vi "TankCommandProcess.vi"(10 "Sensor Cluster":T6, 11 "Command":T8) -> (1 "Non PID Drive Values":T3, 2 "PID Values":T4, 3 "PID Ranges":T1)   [LabVIEW 2017]
uses:
  <userlib>/836-Library/Drive/Drive_Code_V2/Drive_Code_Support/Command_Sends/Drive_Code_Command_Type.ctl
  <userlib>/836-Library/Drive/Drive_Code_V2/Drive_Code_Support/Command_Sends/Drive_Code_Command_List.ctl
  <userlib>/836-Library/Drive/Drive_Code_V2/Drive_Code_Support/SensorTypedefs/Sensor_Cluster.ctl
  <userlib>/836-Library/Drive/Drive_Code_V2/Drive_Code_Support/SensorTypedefs/Camera_Cluster.ctl
  <userlib>/836-Library/Drive/Drive_Code_V2/Drive_Code_Support/PidClusters/DrivePidInputs.ctl
  <userlib>/836-Library/Drive/Drive_Code_V2/Drive_Code_Support/PidClusters/PidInputs.ctl
  <userlib>/836-Library/Drive/Drive_Code_V2/Drive_Code_Support/DriveTrains/Drive_Values.ctl
  <userlib>/836-Library/Drive/Drive_Code_V2/Drive_Code_Support/PidClusters/DrivePidRange.ctl
  <userlib>/836-Library/Drive/Drive_Code_V2/Drive_Code_Support/PidClusters/PidRange.ctl
  <userlib>/836-Library/Drive/Drive_Code_V2/Drive_Code_Support/Command_Sends/CommandTypeInfo/TankDriveParam.ctl
  <userlib>/836-Library/Drive/Drive_Code_V2/Drive_Code_Support/Command_Sends/CommandTypeInfo/DriveContinuousParam.ctl
  <userlib>/836-Library/Drive/Drive_Code_V2/Drive_Code_Support/Command_Sends/CommandTypeInfo/AngleInfo.ctl
  <userlib>/836-Library/Drive/Drive_Code_V2/Drive_Code_Support/Command_Sends/CommandTypeInfo/TurnParam.ctl
  <userlib>/836-Library/Drive/Drive_Code_V2/Drive_Code_Support/Command_Sends/CommandTypeInfo/DriveDistanceParam.ctl
  <userlib>/836-Library/Drive/Drive_Code_V2/Drive_Code_Support/Command_Sends/CommandTypeInfo/DistanceInfo.ctl
  <userlib>/836-Library/Drive/Drive_Code_V2/Drive_Code_Support/Command_Sends/CommandTypeInfo/HoldPositionParam.ctl
  <userlib>/836-Library/Drive/Drive_Code_V2/Drive_Code_Support/Command_Sends/CommandTypeInfo/HoldYawParam.ctl
  <userlib>/836-Library/Drive/Drive_Code_V2/Drive_Code_Support/Command_Sends/CommandTypeInfo/FollowCameraparam.ctl
  <userlib>/836-Library/Drive/Drive_Code_V2/Drive_Code_Support/Command_Sends/CommandTypeInfo/TurnToCameraParam.ctl
  <userlib>/836-Library/Drive/Drive_Code_V2/Drive_Code_Support/Command_Sends/CommandTypeInfo/ApproachCameraParam.ctl
  <userlib>/836-Library/Drive/Drive_Code_V2/Drive_Code_Support/Command_Sends/CommandTypeInfo/CheesyDriveParam.ctl
panel:
  in  "Quick Turn Deadzone":dbl(knob)=0.05 scale=0.0..0.1
  # "I/O"
  # "Configuration Values"
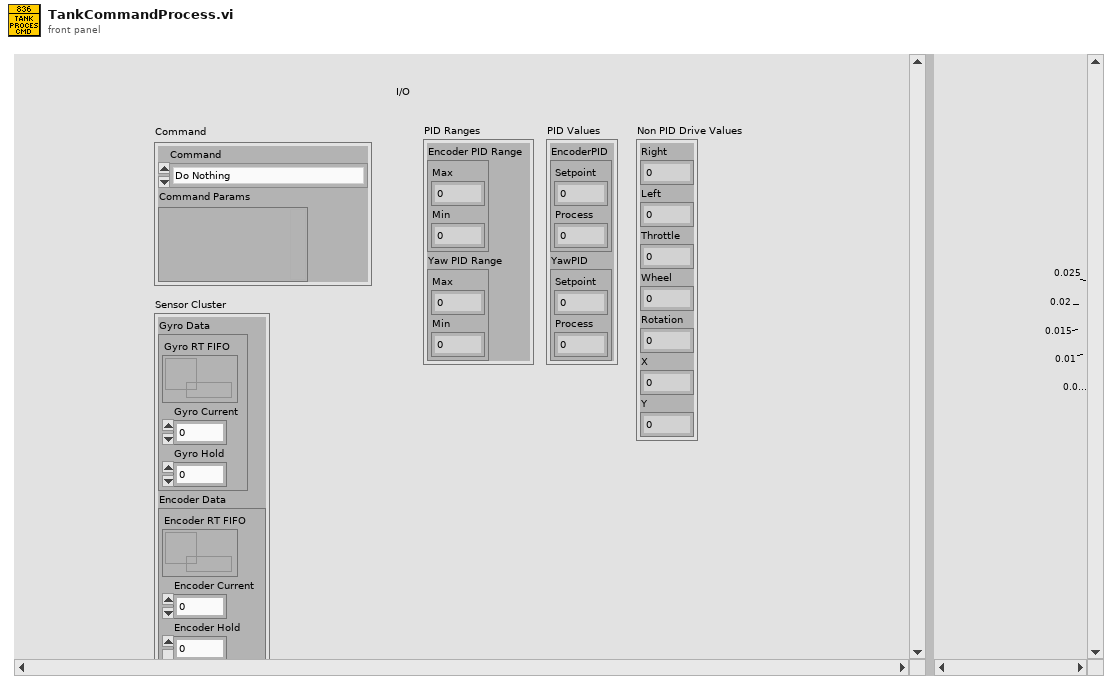
[diagram p1: front panel]
types:
  T1 = typedef "DrivePidRange.ctl" = cluster{"Encoder PID Range":T2, "Yaw PID Range":T2}
  T2 = typedef "PidRange.ctl" = cluster{"Max":dbl, "Min":dbl}
  T3 = typedef "Drive_Values.ctl" = cluster{"Right":dbl, "Left":dbl, "Throttle":dbl, "Wheel":dbl, "Rotation":dbl, "X":dbl, "Y":dbl}
  T4 = typedef "DrivePidInputs.ctl" = cluster{"EncoderPID":T5, "YawPID":T5}
  T5 = typedef "PidInputs.ctl" = cluster{"Setpoint":dbl, "Process":dbl}
  T6 = typedef "Sensor_Cluster.ctl" = cluster{"Gyro Data":cluster{"Gyro RT FIFO":refnum<k33>, "Gyro Current":dbl, "Gyro Hold":dbl}, "Encoder Data":cluster{"Encoder RT FIFO":refnum<k33>, "Encoder Current":dbl, "Encoder Hold":dbl}, "Camera Data":cluster{"Camera RT FIFO":refnum<k33>, "Camera Current":T7}}
  T7 = typedef "Camera_Cluster.ctl" = cluster{" Angle":dbl, "Valid":bool}
  T8 = typedef "Drive_Code_Command_Type.ctl" = cluster{"Command":T9, "Command Params":variant}
  T9 = typedef "Drive_Code_Command_List.ctl" = enum16{"Do Nothing", "Tank Drive", "Drive Continuous", "Turn", "Drive Distance", "Hold Position", "Hold Yaw", "Follow Camera", "Turn to Camera", "Approach Camera", "PID Update", "Cheesy Drive", "Update Period", "Update PID Inversions"}
  T10 = typedef "TankDriveParam.ctl" = cluster{"Left":dbl, "Right":dbl}
  T11 = typedef "DriveContinuousParam.ctl" = cluster{"Max Turn Power":dbl, "Angle To Drive At":T12, "Foward Power":dbl}
  T12 = typedef "AngleInfo.ctl" = cluster{"Angle":dbl, "Angle Absolute?":bool}
  T13 = typedef "TurnParam.ctl" = cluster{"Max Power":dbl, "Angle To Turn To":T12}
  T14 = typedef "DriveDistanceParam.ctl" = cluster{"Max Turn Power":dbl, "Distance To Drive":T15, "Angle To Drive At":T12, "Max Forward Power":dbl}
  T15 = typedef "DistanceInfo.ctl" = cluster{"Distance":dbl, "Distance Absolute?":bool}
  T16 = typedef "HoldPositionParam.ctl" = cluster{"Max Turn Power":dbl, "Max Forward Power":dbl}
  T17 = typedef "HoldYawParam.ctl" = cluster{"Max Turn Power":dbl, "Forward Power":dbl}
  T18 = typedef "FollowCameraparam.ctl" = cluster{"Max Turn Power":dbl, "Forward Power":dbl}
  T19 = typedef "TurnToCameraParam.ctl" = cluster{"Max Turn Power":dbl}
  T20 = typedef "ApproachCameraParam.ctl" = cluster{"Max Turn Power":dbl, "Distance To Drive":T15, "Max Forward Power":dbl}
  T21 = typedef "CheesyDriveParam.ctl" = cluster{"Throttle":dbl, "Wheel":dbl}
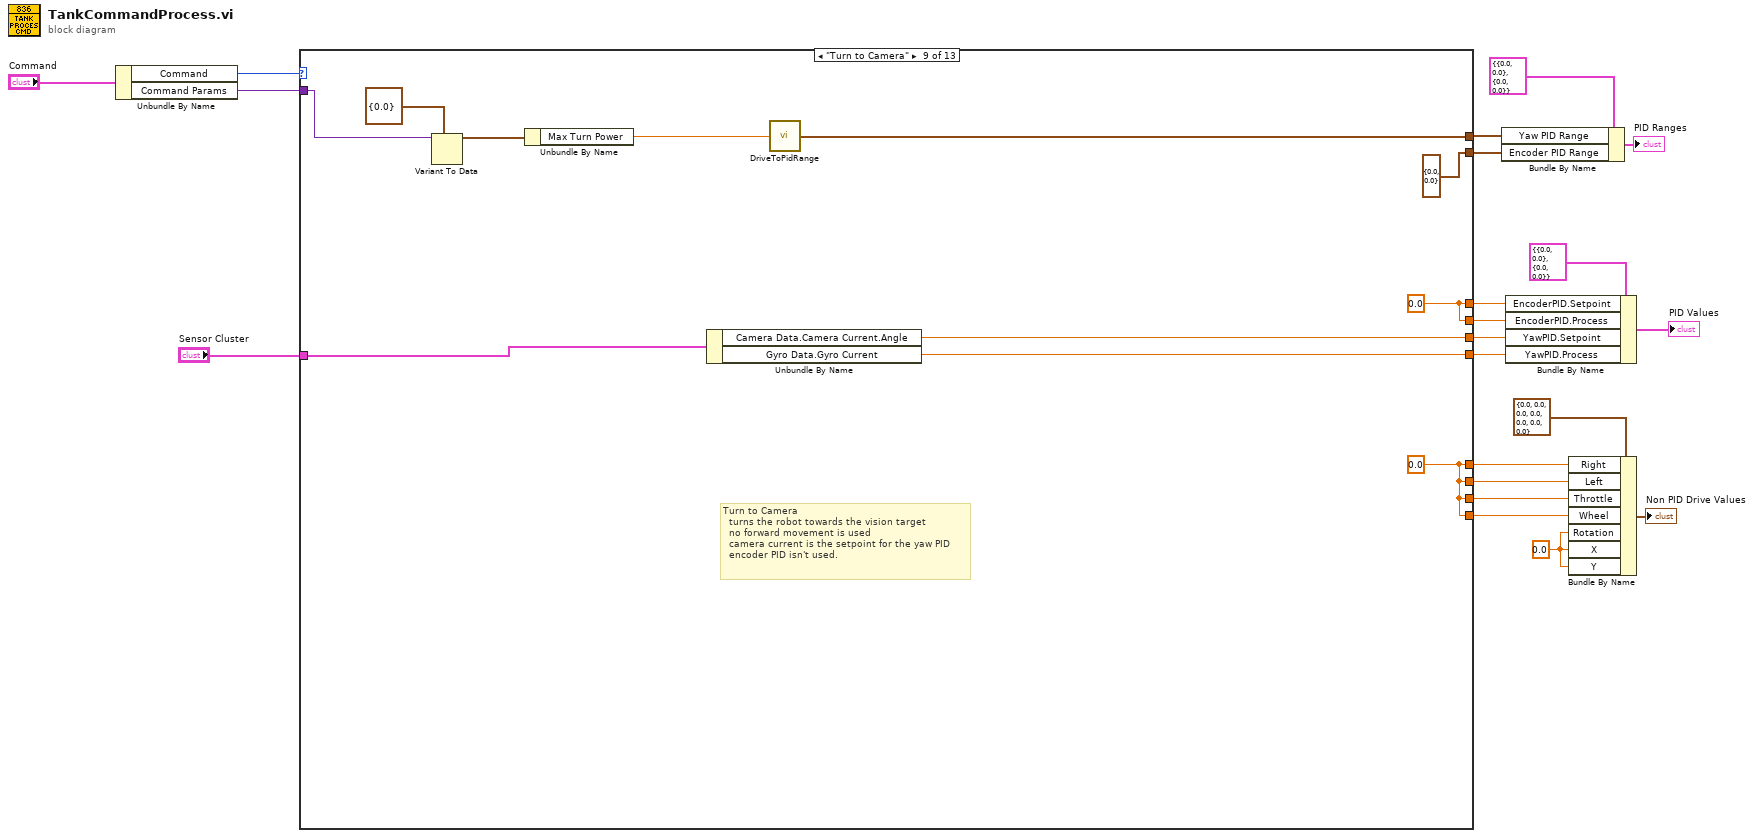
[diagram p0: block diagram]
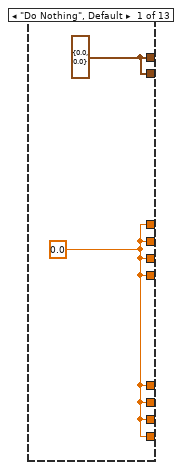
[diagram p2: hidden frame]
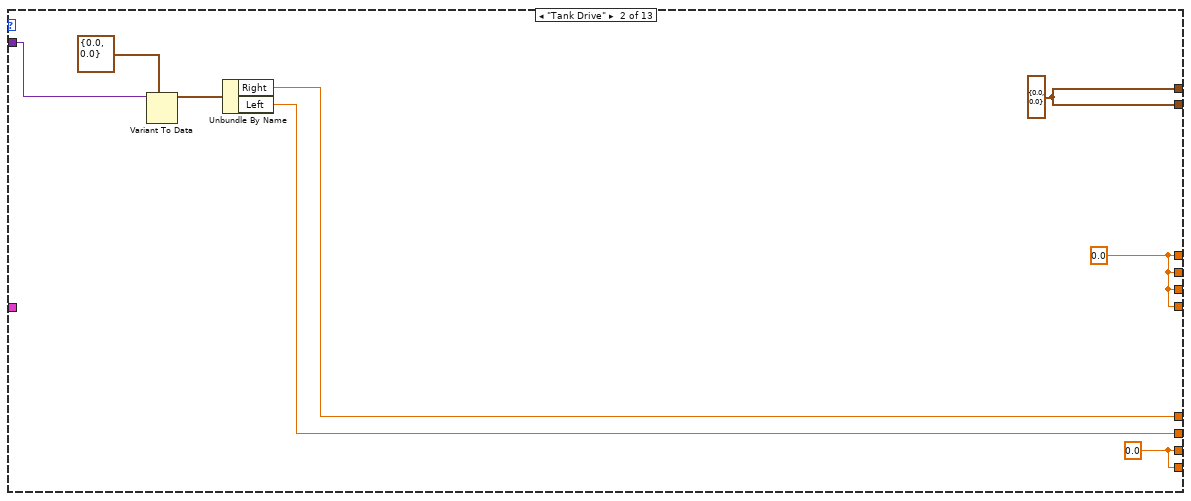
[diagram p3: hidden frame]
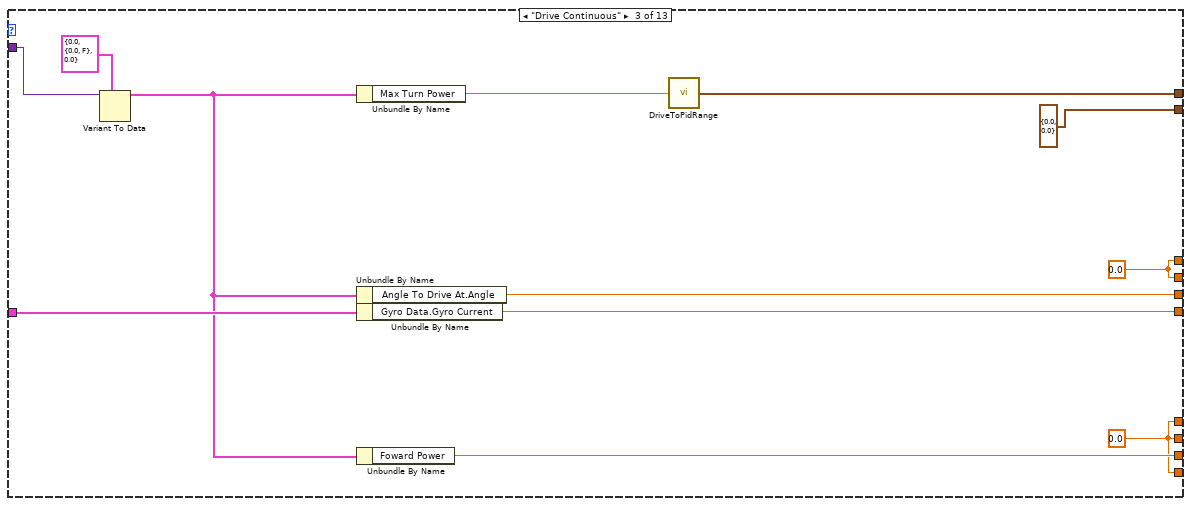
[diagram p4: hidden frame]
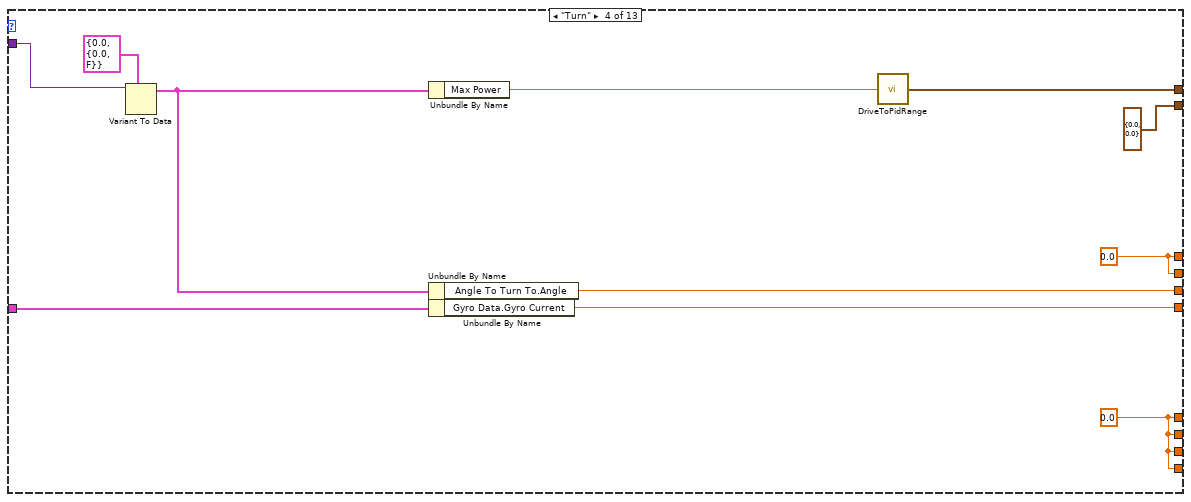
[diagram p5: hidden frame]
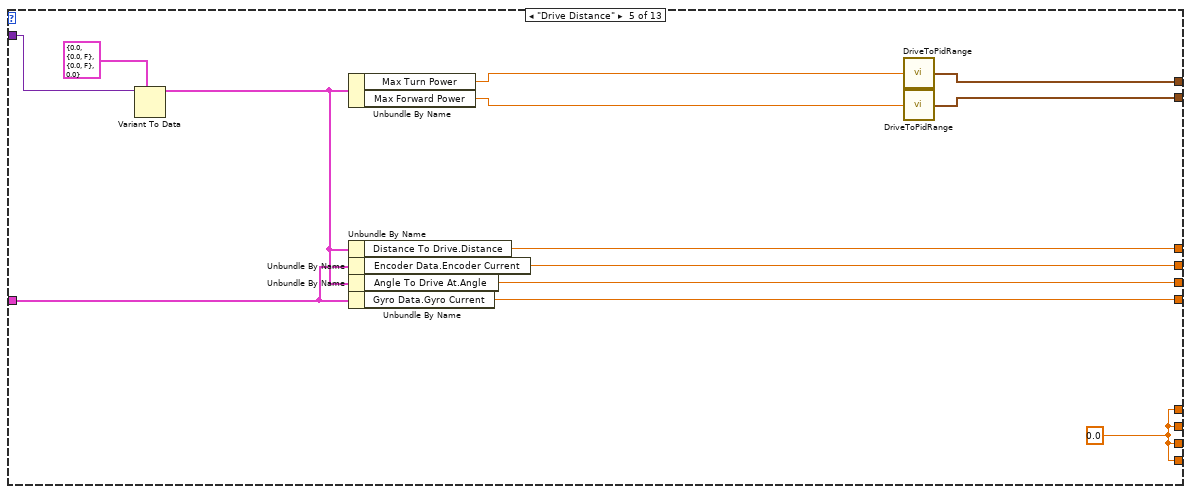
[diagram p6: hidden frame]
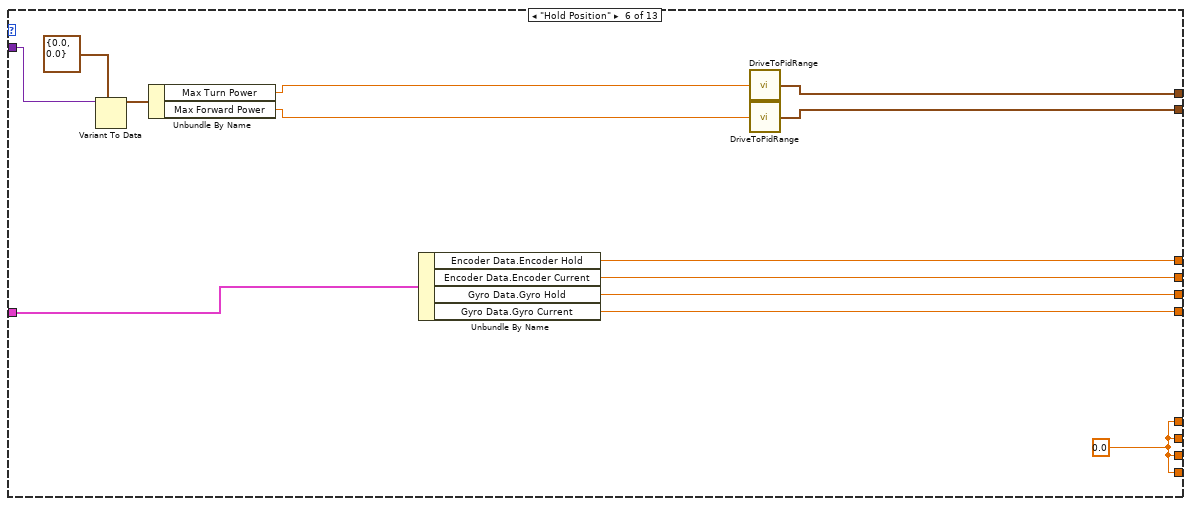
[diagram p7: hidden frame]
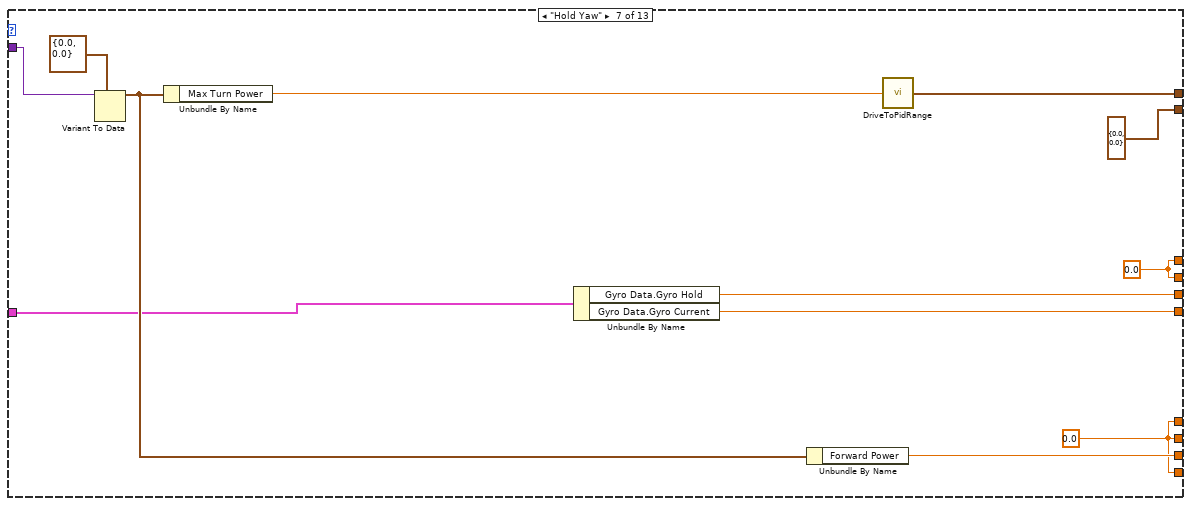
[diagram p8: hidden frame]
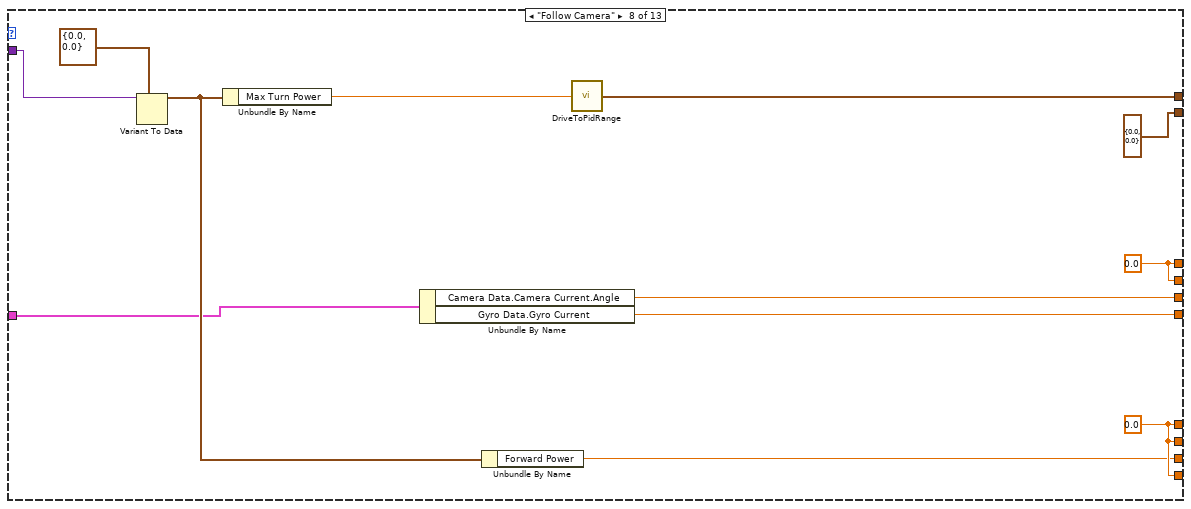
[diagram p9: hidden frame]
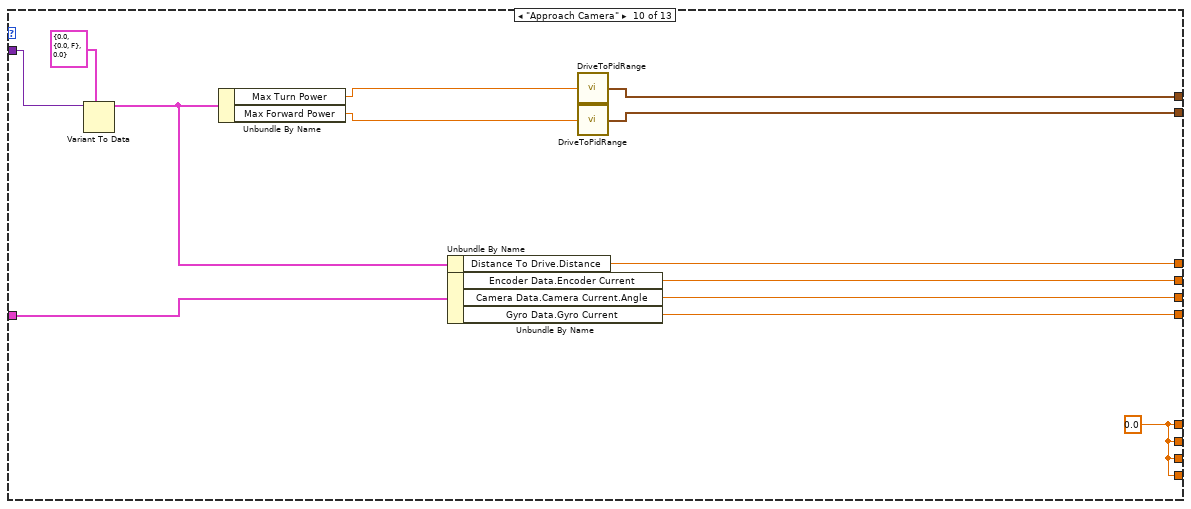
[diagram p10: hidden frame]
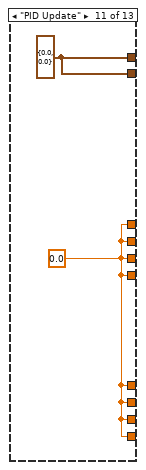
[diagram p11: hidden frame]
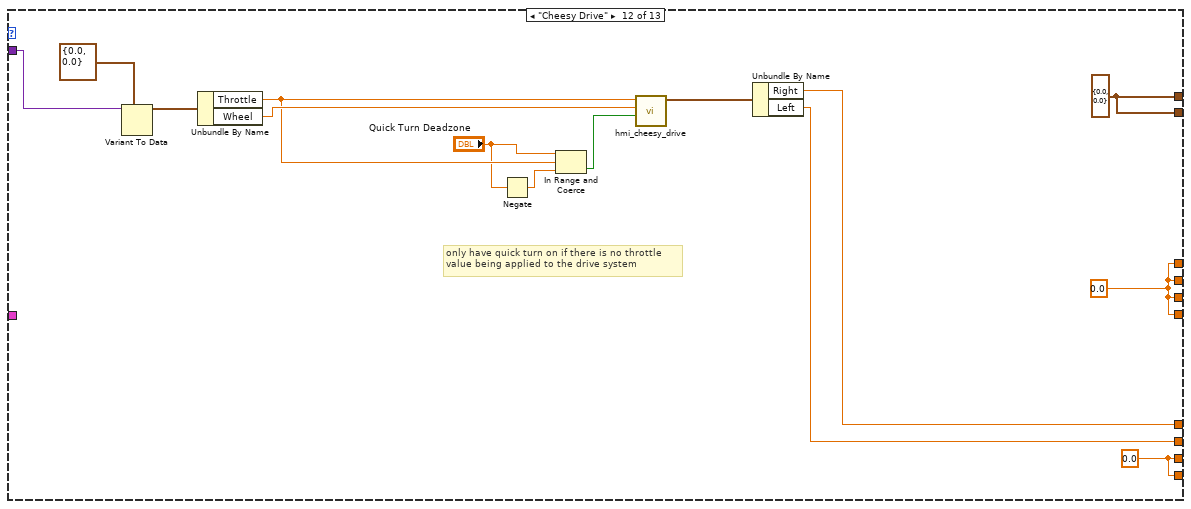
[diagram p12: hidden frame]
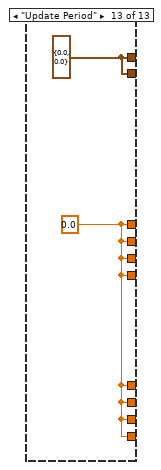
[diagram p13: hidden frame]
diagram:
  w8 = 0.0 ("Rotation")
  n1 = Unbundle By Name("Command") -> ("Command"=w20:T9, "Command Params"=w19:variant)
  n2 = case shown="\"Turn to Camera\"" w20 {
    tunnel: w19 -> [_ w30 w42 w51 w67 w80 w92 w104 w115 w128 _ w143 _]
    tunnel: "Sensor Cluster" -> [_ _ w43 w47 w60 w72 w83 w95 w107 w120 _ _ _]
    tunnel: [w22 w31 w36 w53 w59 w71 w87 w99 w108 w119 w129 w144 w145] -> w16
    tunnel: [w22 w31 w36 w53 w58 w70 w87 w99 w108 w118 w129 w144 w145] -> w15
    tunnel: [w22 w31 w38 w44 w57 w69 w82 w94 w106 w117 w129 w144 w145] -> w14
    tunnel: [w22 w31 w37 w46 w56 w68 w81 w93 w105 w116 w129 w144 w145] -> w13
    tunnel: [w22 w27 w33 w54 w55 w73 w88 w98 w109 w122 w129 w139 w145] -> w10
    tunnel: [w22 w26 w33 w54 w55 w73 w88 w98 w109 w122 w129 w138 w145] -> w9
    tunnel: [w23 w25 w40 w49 w63 w74 w85 w101 w111 w124 w130 w132 w146] -> w3
    tunnel: [w22 w24 w34 w54 w55 w73 w89 w96 w109 w122 w129 w131 w145] -> w6
    tunnel: [w22 w24 w33 w54 w55 w73 w88 w98 w109 w122 w129 w131 w145] -> w5
    tunnel: [w23 w25 T2 {"Max"=0.0, "Min"=0.0} ("PID Range") T2 {"Max"=0.0, "Min"=0.0} ("PID Range") w62 w75 T2 {"Max"=0.0, "Min"=0.0} ("PID Range") T2 {"Max"=0.0, "Min"=0.0} ("PID Range") T2 {"Max"=0.0, "Min"=0.0} ("PID Range") w123 w130 w132 w146] -> w2
    frame "Do Nothing", Default {
      w23 = T2 {"Max"=0.0, "Min"=0.0} ("PID Range")
      w22 = 0.0
    }
    frame "Tank Drive" {
      w24 = 0.0 ("Encoder Hold")
      w25 = T2 {"Max"=0.0, "Min"=0.0} ("PID Range")
      w31 = 0.0
      n3 = Variant To Data(type=T10 {"Left"=0.0, "Right"=0.0} ("Tank Drive Param"), Variant=w30) -> (data=w28:T10)  [unwired: 1 in, 1 out]
      n4 = Unbundle By Name(w28) -> ("Right"=w27:dbl, "Left"=w26:dbl)
    }
    frame "Drive Continuous" {
      w33 = 0.0
      w36 = 0.0
      n5 = Variant To Data(type=T11 {"Max Turn Power"=0.0, "Angle To Drive At"={"Angle"=0.0, "Angle Absolute?"=FALSE}, "Foward Power"=0.0} ("Drive Continuous Param"), Variant=w42) -> (data=w35:T11)  [unwired: 1 in, 1 out]
      n6 = Unbundle By Name(w35) -> ("Max Turn Power"=w39:dbl)
      n7 = Unbundle By Name(w35) -> ("Angle To Drive At.Angle"=w38:dbl)
      n8 = Unbundle By Name(w43) -> ("Gyro Data.Gyro Current"=w37:dbl)
      n9 = Unbundle By Name(w35) -> ("Foward Power"=w34:dbl)
      n10 = call <userlib>:"DriveToPidRange.vi"("Max Power"=w39) -> ("PID Range"=w40:T2)
    }
    frame "Turn" {
      w53 = 0.0
      w54 = 0.0 ("Right")
      n11 = Variant To Data(type=T13 {"Max Power"=0.0, "Angle To Turn To"={"Angle"=0.0, "Angle Absolute?"=FALSE}} ("Turn Param"), Variant=w51) -> (data=w45:T13)  [unwired: 1 in, 1 out]
      n12 = Unbundle By Name(w45) -> ("Max Power"=w48:dbl)
      n13 = Unbundle By Name(w45) -> ("Angle To Turn To.Angle"=w44:dbl)
      n14 = Unbundle By Name(w47) -> ("Gyro Data.Gyro Current"=w46:dbl)
      n15 = call <userlib>:"DriveToPidRange.vi"("Max Power"=w48) -> ("PID Range"=w49:T2)
    }
    frame "Drive Distance" {
      w55 = 0.0
      n16 = Variant To Data(type=T14 {"Max Turn Power"=0.0, "Distance To Drive"={"Distance"=0.0, "Distance Absolute?"=FALSE}, "Angle To Drive At"={"Angle"=0.0, "Angle Absolute?"=FALSE}, "Max Forward Power"=0.0} ("Drive Distance Param"), Variant=w67) -> (data=w61:T14)  [unwired: 1 in, 1 out]
      n17 = Unbundle By Name(w61) -> ("Max Turn Power"=w64:dbl, "Max Forward Power"=w65:dbl)
      n18 = Unbundle By Name(w61) -> ("Distance To Drive.Distance"=w59:dbl)
      n19 = Unbundle By Name(w60) -> ("Encoder Data.Encoder Current"=w58:dbl)
      n20 = Unbundle By Name(w61) -> ("Angle To Drive At.Angle"=w57:dbl)
      n21 = Unbundle By Name(w60) -> ("Gyro Data.Gyro Current"=w56:dbl)
      n22 = call <userlib>:"DriveToPidRange.vi"("Max Power"=w64) -> ("PID Range"=w63:T2)
      n23 = call <userlib>:"DriveToPidRange.vi"("Max Power"=w65) -> ("PID Range"=w62:T2)
    }
    frame "Hold Position" {
      w73 = 0.0 ("Right")
      n24 = Variant To Data(type=T16 {"Max Turn Power"=0.0, "Max Forward Power"=0.0} ("Hold Position Param"), Variant=w80) -> (data=w78:T16)  [unwired: 1 in, 1 out]
      n25 = Unbundle By Name(w78) -> ("Max Turn Power"=w77:dbl, "Max Forward Power"=w76:dbl)
      n26 = Unbundle By Name(w72) -> ("Encoder Data.Encoder Hold"=w71:dbl, "Encoder Data.Encoder Current"=w70:dbl, "Gyro Data.Gyro Hold"=w69:dbl, "Gyro Data.Gyro Current"=w68:dbl)
      n27 = call <userlib>:"DriveToPidRange.vi"("Max Power"=w77) -> ("PID Range"=w74:T2)
      n28 = call <userlib>:"DriveToPidRange.vi"("Max Power"=w76) -> ("PID Range"=w75:T2)
    }
    frame "Hold Yaw" {
      w87 = 0.0 ("Encoder Hold")
      w88 = 0.0
      n29 = Variant To Data(type=T17 {"Max Turn Power"=0.0, "Forward Power"=0.0} ("Hold Yaw Param"), Variant=w92) -> (data=w90:T17)  [unwired: 1 in, 1 out]
      n30 = Unbundle By Name(w90) -> ("Max Turn Power"=w84:dbl)
      n31 = Unbundle By Name(w83) -> ("Gyro Data.Gyro Hold"=w82:dbl, "Gyro Data.Gyro Current"=w81:dbl)
      n32 = Unbundle By Name(w90) -> ("Forward Power"=w89:dbl)
      n33 = call <userlib>:"DriveToPidRange.vi"("Max Power"=w84) -> ("PID Range"=w85:T2)
    }
    frame "Follow Camera" {
      w98 = 0.0 ("Encoder Hold")
      w99 = 0.0 ("Encoder Hold")
      n34 = Variant To Data(type=T18 {"Max Turn Power"=0.0, "Forward Power"=0.0} ("Follow Camera Param"), Variant=w104) -> (data=w97:T18)  [unwired: 1 in, 1 out]
      n35 = Unbundle By Name(w97) -> ("Max Turn Power"=w102:dbl)
      n36 = Unbundle By Name(w95) -> ("Camera Data.Camera Current.Angle"=w94:dbl, "Gyro Data.Gyro Current"=w93:dbl)
      n37 = Unbundle By Name(w97) -> ("Forward Power"=w96:dbl)
      n38 = call <userlib>:"DriveToPidRange.vi"("Max Power"=w102) -> ("PID Range"=w101:T2)
    }
    frame "Turn to Camera" {
      w108 = 0.0 ("Encoder Hold")
      w109 = 0.0 ("Encoder Hold")
      # "Turn to Camera\n  turns the robot towards the vision target\n  no forward movement is used\n  camera current is the setpoint for the yaw PID\n  encoder PID isn't used."
      n39 = Variant To Data(type=T19 {"Max Turn Power"=0.0} ("Turn To Camera Param"), Variant=w115) -> (data=w113:T19)  [unwired: 1 in, 1 out]
      n40 = Unbundle By Name(w113) -> ("Max Turn Power"=w112:dbl)
      n41 = Unbundle By Name(w107) -> ("Camera Data.Camera Current.Angle"=w106:dbl, "Gyro Data.Gyro Current"=w105:dbl)
      n42 = call <userlib>:"DriveToPidRange.vi"("Max Power"=w112) -> ("PID Range"=w111:T2)
    }
    frame "Approach Camera" {
      w122 = 0.0 ("Encoder Hold")
      n43 = Variant To Data(type=T20 {"Max Turn Power"=0.0, "Distance To Drive"={"Distance"=0.0, "Distance Absolute?"=FALSE}, "Max Forward Power"=0.0} ("Approach Camera Param"), Variant=w128) -> (data=w121:T20)  [unwired: 1 in, 1 out]
      n44 = Unbundle By Name(w121) -> ("Max Turn Power"=w126:dbl, "Max Forward Power"=w125:dbl)
      n45 = Unbundle By Name(w121) -> ("Distance To Drive.Distance"=w119:dbl)
      n46 = Unbundle By Name(w120) -> ("Encoder Data.Encoder Current"=w118:dbl, "Camera Data.Camera Current.Angle"=w117:dbl, "Gyro Data.Gyro Current"=w116:dbl)
      n47 = call <userlib>:"DriveToPidRange.vi"("Max Power"=w126) -> ("PID Range"=w124:T2)
      n48 = call <userlib>:"DriveToPidRange.vi"("Max Power"=w125) -> ("PID Range"=w123:T2)
    }
    frame "PID Update" {
      w130 = T2 {"Max"=0.0, "Min"=0.0} ("PID Range")
      w129 = 0.0
    }
    frame "Cheesy Drive" {
      w131 = 0.0 ("Foward Power")
      w132 = T2 {"Max"=0.0, "Min"=0.0} ("PID Range")
      w144 = 0.0
      # "only have quick turn on if there is no throttle\nvalue being applied to the drive system"
      n49 = Variant To Data(type=T21 {"Throttle"=0.0, "Wheel"=0.0} ("Cheesy Drive Param"), Variant=w143) -> (data=w141:T21)  [unwired: 1 in, 1 out]
      n50 = Unbundle By Name(w141) -> ("Throttle"=w136:dbl, "Wheel"=w137:dbl)
      n51 = Negate(x="Quick Turn Deadzone") -> (-x=w134:dbl)
      n52 = In Range and Coerce(upper limit="Quick Turn Deadzone", x=w136, lower limit=w134) -> (In Range?=w133:bool)  [unwired: 1 out]
      n53 = call <userlib>:"hmi_cheesy_drive.vi"("Quick Turn"=w133, "Wheel"=w137, "Throttle"=w136) -> ("Drive Data"=w140:cluster{"Left":dbl, "Right":dbl})  [unwired: 8 in]
      n54 = Unbundle By Name(w140) -> ("Right"=w139:dbl, "Left"=w138:dbl)
    }
    frame "Update Period" {
      w145 = 0.0 ("Encoder Hold")
      w146 = T2 {"Max"=0.0, "Min"=0.0} ("PID Range")
    }
  }
  n55 = Bundle By Name(cluster=T1 {"Encoder PID Range"={"Max"=0.0, "Min"=0.0}, "Yaw PID Range"={"Max"=0.0, "Min"=0.0}} ("Drive PID Ranges"), "Yaw PID Range"=w3, "Encoder PID Range"=w2) -> (→"PID Ranges":T1)
  n56 = Bundle By Name(cluster=T4 {"EncoderPID"={"Setpoint"=0.0, "Process"=0.0}, "YawPID"={"Setpoint"=0.0, "Process"=0.0}} ("DrivePidInputs"), "EncoderPID.Setpoint"=w16, "EncoderPID.Process"=w15, "YawPID.Setpoint"=w14, "YawPID.Process"=w13) -> (→"PID Values":T4)
  n57 = Bundle By Name(cluster=T3 {"Right"=0.0, "Left"=0.0, "Throttle"=0.0, "Wheel"=0.0, "Rotation"=0.0, "X"=0.0, "Y"=0.0} ("Drive Values"), "Right"=w10, "Left"=w9, "Throttle"=w6, "Wheel"=w5, "Rotation"=w8, "X"=w8, "Y"=w8) -> (→"Non PID Drive Values":T3)
